vi "Read Valid Registration Types.vi"(11 "EventHandler Type":refnum<class "ListboxEventHandler.lvclass">) -> (2 "Valid Registration Types":T1[](array[typedef]))   [LabVIEW 2017, in "ActorEvents.lvlib" / "ListboxEventHandler.lvclass"]
uses:
  <vilib>/gpm_packages/@cs/mva-viewable/Source/ActorEvents/EventHandler/ListboxEventHandler/ListboxEventHandler.lvclass
  <vilib>/event_ctls.llb/lveventtype.ctl
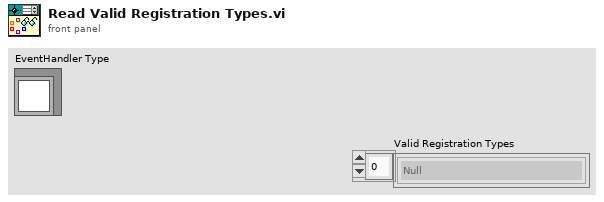
[diagram p1: front panel]
types:
  T1 = typedef "lveventtype.ctl" = enum32{"Null", "Timeout", "Annotation Menu Selection", "Annotation Menu Selection?", "App Instance Close", "App Instance Close?", "Autoscale Range Change", "Bookmark Info Change", "Cell Edit", "Cell Edit?", "Cursor Grab", "Cursor Grab?", "Cursor Menu Selection", "Cursor Menu Selection?", "Cursor Move", "Cursor Release", "Data Change", "Direction Change", "Display State Change", "Drag Ended", "Drag Enter", "Drag Leave", "Drag Over", "Drag Source Update", "Drag Starting", "Drag Starting?", "Drop", "Exec State Change", "Key Down", "Key Down?", "Key Repeat", "Key Repeat?", "Key Up", "Listbox Double Click", "Menu Activation?", "Menu Selection (App)", "Menu Selection? (App)", "Menu Selection (User)", "Mouse Down", "Mouse Down?", "Mouse Enter", "Mouse Leave", "Mouse Move", "Mouse Up", "Mouse Wheel", "NI Security User Change (App)", "Pane Size", "Panel Close", "Panel Close?", "Panel Resize", "Plot Attribute Change", "Scale Range Change", "Shortcut Menu Activation?", "Shortcut Menu Selection (App)", "Shortcut Menu Selection? (App)", "Shortcut Menu Selection (User)", "Tree Double Click", "Tree Drag", "Tree Drag?", "Tree Drop", "Tree Drop?", "Tree Item Close", "Tree Item Close?", "Tree Item Open", "Tree Item Open?", "User Event", "Value Change"}
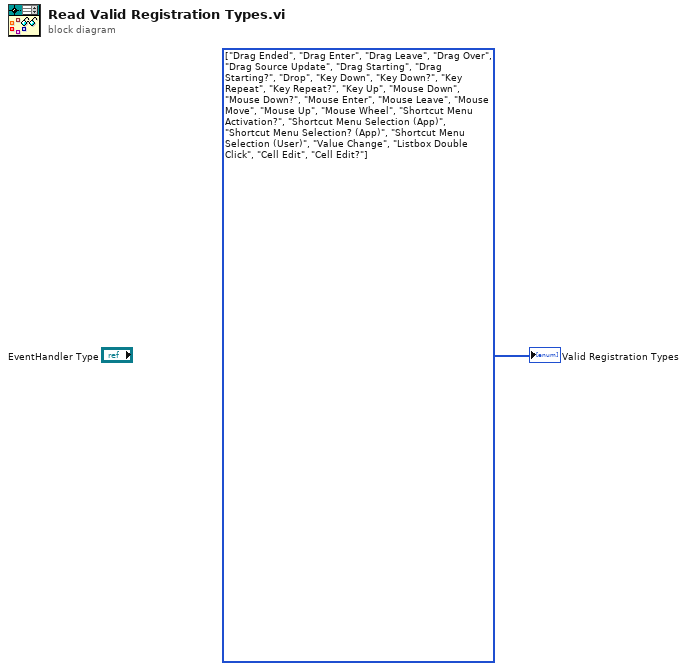
[diagram p0: block diagram]
diagram:
  w1 = T1[] [enum."Drag Ended", enum."Drag Enter", enum."Drag Leave", enum."Drag Over", enum."Drag Source Update", enum."Drag Starting", enum."Drag Starting?", enum."Drop", enum."Key Down", enum."Key Down?", enum."Key Repeat", enum."Key Repeat?", enum."Key Up", enum."Mouse Down", enum."Mouse Down?", enum."Mouse Enter", enum."Mouse Leave", enum."Mouse Move", enum."Mouse Up", enum."Mouse Wheel", enum."Shortcut Menu Activation?", enum."Shortcut Menu Selection (App)", enum."Shortcut Menu Selection? (App)", enum."Shortcut Menu Selection (User)", enum."Value Change", enum."Listbox Double Click", enum."Cell Edit", enum."Cell Edit?"] items=["Null", "Timeout", "Annotation Menu Selection", "Annotation Menu Selection?", "App Instance Close", "App Instance Close?", "Autoscale Range Change", "Bookmark Info Change", "Cell Edit", "Cell Edit?", "Cursor Grab", "Cursor Grab?", "Cursor Menu Selection", "Cursor Menu Selection?", "Cursor Move", "Cursor Release", "Data Change", "Direction Change", "Display State Change", "Drag Ended", "Drag Enter", "Drag Leave", "Drag Over", "Drag Source Update", "Drag Starting", "Drag Starting?", "Drop", "Exec State Change", "Key Down", "Key Down?", "Key Repeat", "Key Repeat?", "Key Up", "Listbox Double Click", "Menu Activation?", "Menu Selection (App)", "Menu Selection? (App)", "Menu Selection (User)", "Mouse Down", "Mouse Down?", "Mouse Enter", "Mouse Leave", "Mouse Move", "Mouse Up", "Mouse Wheel", "NI Security User Change (App)", "Pane Size", "Panel Close", "Panel Close?", "Panel Resize", "Plot Attribute Change", "Scale Range Change", "Shortcut Menu Activation?", "Shortcut Menu Selection (App)", "Shortcut Menu Selection? (App)", "Shortcut Menu Selection (User)", "Tree Double Click", "Tree Drag", "Tree Drag?", "Tree Drop", "Tree Drop?", "Tree Item Close", "Tree Item Close?", "Tree Item Open", "Tree Item Open?", "User Event", "Value Change"] ("Valid Registration Types")
  "Valid Registration Types" <- w1
